vi "3458 read meas .vi"(2 "error in":errorcluster, 4 "address string":string) -> (0 "error out":errorcluster, 1 "data":string)   [LabVIEW 2014]
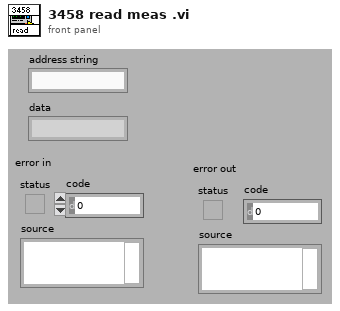
[diagram p1: front panel]
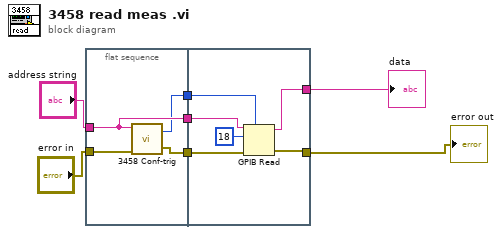
[diagram p0: block diagram]
diagram:
  n1 = flat-sequence {
    tunnel: "error in" -> [w11]
    tunnel: "address string" -> [w10]
    tunnel: [w10] -> w3
    tunnel: [w9] -> w2
    tunnel: [w8] -> w1
    tunnel: [w14] -> w4
    tunnel: [w16] -> w5
    tunnel: w3 -> [w15]
    tunnel: w2 -> [w13]
    tunnel: w1 -> [w12]
    frame #0 {
      n2 = call "3458 Conf-trig.vi"("error in"=w11, "address string"=w10) -> ("error out"=w9:errorcluster, "timeout ms (488.2 global)"=w8:i32)  [unwired: 2 in]
    }
    frame #1 {
      n3 = GPIB Read(0:w15, 1:18 ("byte count"), 3:w13, 4:w12) -> (5:w16:string, 7:w14:errorcluster)  [unwired: 1 in, 1 out]
    }
  }
  "data" <- w5
  "error out" <- w4
